vi "START CHECK OUT ITEMS.vi"(11 "REFERENCES":T1) -> ()   [LabVIEW 2019]
uses:
  Controls/References Cluster.ctl
  <vilib>/userDefined/High Color/IMAQdx.ctl
  Controls/Custom Calendar/Custom Calendar.xctl
  <vilib>/Utility/miscctls.llb/LVRowAndColumnTypeDef.ctl
types:
  T1 = typedef "References Cluster.ctl" = cluster{"MAIN PAGES":refnum<vi>, "ADD/EDIT ITEM REFERENCES":cluster{"Identifier":refnum<vi>, "BYU ICN #":refnum<vi>, "Item Description":refnum<vi>, "Comments":refnum<vi>, "Checked Out Date":refnum<vi>, "Due Date":refnum<vi>, "Check Out Location":refnum<vi>, "Reminder Count":refnum<vi>, "Most Recent Reminder Date":refnum<vi>, "BYU ID #":refnum<vi>, "Building/Room":refnum<vi>, "Location in Room":refnum<vi>, "Manual":refnum<vi>, "Manufacturer":refnum<vi>, "Model #":refnum<vi>, "Serial #":refnum<vi>, "Date Acquired":refnum<vi>, "ADD/EDIT ITEM LABEL":refnum<vi>, "ARCHIVE ITEM":refnum<vi>, "Archive Item Inputs":refnum<vi>, "Reminder Notes":refnum<vi>}, "ADD/EDIT USER REFERENCES":cluster{"BYU ID # (##-###-####)":refnum<vi>, "First Name":refnum<vi>, "Last Name":refnum<vi>, "Phone Number (###-###-####)":refnum<vi>, "Email":refnum<vi>, "Department":refnum<vi>, "Graduation Status":refnum<vi>, "Anticipated Graduation Year":refnum<vi>, "Credit Score":refnum<vi>, "Date Added":refnum<vi>, "Graduation Clearance Date":refnum<vi>, "Picture File Name":refnum<vi>, "ADD/EDIT USER LABEL":refnum<vi>, "Department Map":refnum<vi>, "Status Map":refnum<vi>, "Anticipated Graduation Year Map":refnum<vi>, "User Agreement":refnum<vi>, "User Comments":refnum<vi>, "Camera":refnum<vi>}, "RETURN ITEM REFERENCES":cluster{"Item or Person:":refnum<vi>, "Search Return Results":refnum<vi>, "What are you searching for?":refnum<vi>}, "SEARCH DATABASE REFERENCES":cluster{"What to Search For:":refnum<vi>, "Where to Search":refnum<vi>, "Column to Search In":refnum<vi>, "Column to Sort By":refnum<vi>, "Search Database Results":refnum<vi>, "Inventory Column Selector":refnum<vi>, "User Column Selector":refnum<vi>, "Inventory Archive Column Selector":refnum<vi>, "User Archive Column Selector":refnum<vi>, "Sales Tracking Column Selector":refnum<vi>, "Checked In Archive Column Selector":refnum<vi>, "Restore User":refnum<vi>, "Date Range":refnum<vi>, "Dates Less Than":refnum<vi>, "Dates Greater Than":refnum<vi>, "Search Print Receipt":refnum<vi>, "Edit Sale Description":refnum<vi>}, "USER ITEMS REFERENCES":cluster{"USER'S INFORMATION":refnum<vi>, "User's Checked Out Items":refnum<vi>, "User Info Comments":refnum<vi>, "SEE USER INFO COMMENTS":refnum<vi>}, "EDIT ITEMS REFERENCES":cluster{"New Check Out Location":refnum<vi>, "Items to Edit":refnum<vi>, "Edit Items Due Date":refnum<vi>, "New Reminder Notes":refnum<vi>, "New Item Description":refnum<vi>}, "CHECK OUT ITEMS REFERENCES":cluster{"Enter Item:":refnum<vi>, "Check Out Items Due Date":refnum<vi>, "Check Out Location":refnum<vi>, "Items to be Checked Out":refnum<vi>, "Possible Items":refnum<vi>}, "TRANSFER ITEMS REFERENCES":cluster{"Search Parameter":refnum<vi>, "What to Match":refnum<vi>, "Matching Individuals":refnum<vi>, "Items to be Transferred":refnum<vi>}, "SETTINGS REFERENCES":cluster{"PSC Database Settings":refnum<vi>, "PSC Sales Item Spreadsheet":refnum<vi>}, "PSC SALES REFERENCES":cluster{"BYU ID CARD #":refnum<vi>, "Sale Description":refnum<vi>, "Scan or Enter Item Name":refnum<vi>, "Items to be Sold":refnum<vi>, "Grand Total":refnum<vi>, "Item List":refnum<vi>}}
  T2 = typedef "LVRowAndColumnTypeDef.ctl" = cluster{"Row":i32, "Column":i32}
  T3 = enum32{"IDLE", "ADD/EDIT USER", "ADD/EDIT ITEM", "RETURN ITEMS", "SEARCH DATABASE", "USER ITEMS", "CHECK OUT ITEMS", "EDIT ITEMS", "TRANSFER ITEMS", "PSC SALES", "ATRIUM", "INVENTORY TRACKING", "SETTINGS"}
  T4 = cluster{"Enter Item:":refnum<vi>, "Check Out Items Due Date":refnum<vi>, "Check Out Location":refnum<vi>, "Items to be Checked Out":refnum<vi>, "Possible Items":refnum<vi>}
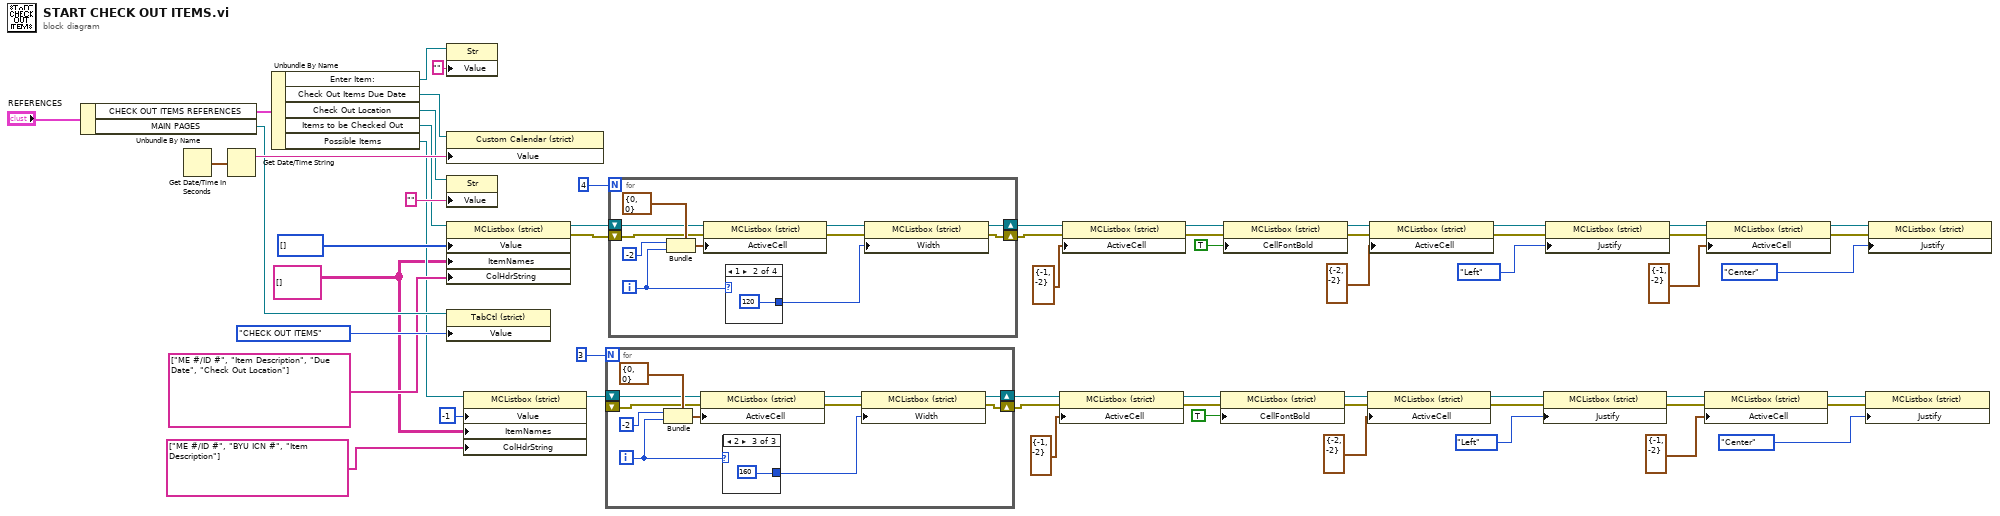
[diagram p0: block diagram]
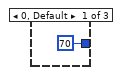
[diagram p2: hidden frame]
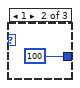
[diagram p3: hidden frame]
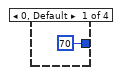
[diagram p4: hidden frame]
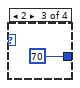
[diagram p5: hidden frame]
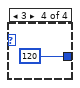
[diagram p6: hidden frame]
diagram:
  w3 = string[][] [] ("Item Names")
  n1 = Unbundle By Name("REFERENCES") -> ("CHECK OUT ITEMS REFERENCES"=w59:T4, "MAIN PAGES"=w49:refnum<vi>)
  n2 = Get Date/Time In Seconds() -> (seconds since 1Jan1904=w55:timestamp)
  n3 = Get Date/Time String(seconds (now)=w55) -> (date string=w54:string)  [unwired: 2 in, 1 out]
  n4 = Unbundle By Name(w59) -> ("Enter Item:"=w58:refnum<vi>, "Check Out Items Due Date"=w56:refnum<vi>, "Check Out Location"=w53:refnum<vi>, "Items to be Checked Out"=w51:refnum<vi>, "Possible Items"=w4:refnum<vi>)
  n5 = property class="Str"(reference=w58, "Value"="") -> ()  [unwired: 1 in, 2 out]
  n6 = property class="Custom Calendar (strict)"(reference=w56, "Value"=w54) -> ()  [unwired: 1 in, 2 out]
  n7 = property class="Str"(reference=w53, "Value"="") -> ()  [unwired: 1 in, 2 out]
  n8 = property class="MCListbox (strict)"(reference=w51, "Value"=i32[] [], "ItemNames"=w3, "ColHdrString"=string[] ["ME #/ID #", "Item Description", "Due Date", "Check Out Location"] ("Column Header Strings[]")) -> (reference out=w46:refnum<vi>, error out=w45:errorcluster)  [unwired: 1 in]
  n9 = property class="TabCtl (strict)"(reference=w49, "Value"=T3."CHECK OUT ITEMS") -> ()  [unwired: 1 in, 2 out]
  n10 = property class="MCListbox (strict)"(reference=w4, "Value"=-1, "ItemNames"=w3, "ColHdrString"=string[] ["ME #/ID #", "BYU ICN #", "Item Description"] ("Column Header Strings[]")) -> (reference out=w5:refnum<vi>)  [unwired: 1 in, 1 out]
  n11 = for {
    N: 3 -> [_]
    shift-right: [w70] -> w24
    shift-left: w5 -> [w67]
    shift-right: [w69] -> w23
    shift-left: _ -> [w66]
    i -> [w63]
    n12 = Bundle(cluster=T2 {"Row"=0, "Column"=0} ("Active Cell:Active Cell"), "Row"=-2, "Column"=w63) -> (w65:T2)
    n13 = property class="MCListbox (strict)"(reference=w67, error in=w66, "ActiveCell"=w65) -> (reference out=w61:refnum<vi>, error out=w60:errorcluster)
    n14 = case shown="2" w63 {
      tunnel: [u32 70 ("Active Cell:Cell Size:Width") u32 100 ("Active Cell:Cell Size:Width") u32 160 ("Active Cell:Cell Size:Width")] -> w62
      frame 0, Default {
      }
      frame 1 {
      }
      frame 2 {
      }
    }
    n15 = property class="MCListbox (strict)"(reference=w61, error in=w60, "Width"=w62) -> (reference out=w70:refnum<vi>, error out=w69:errorcluster)
  }
  n16 = for {
    N: 4 -> [_]
    shift-right: [w84] -> w26
    shift-left: w46 -> [w81]
    shift-right: [w83] -> w27
    shift-left: w45 -> [w80]
    i -> [w77]
    n17 = Bundle(cluster=T2 {"Row"=0, "Column"=0} ("Active Cell:Active Cell"), "Row"=-2, "Column"=w77) -> (w79:T2)
    n18 = property class="MCListbox (strict)"(reference=w81, error in=w80, "ActiveCell"=w79) -> (reference out=w75:refnum<vi>, error out=w74:errorcluster)
    n19 = case shown="1" w77 {
      tunnel: [u32 70 ("Active Cell:Cell Size:Width") u32 120 ("Active Cell:Cell Size:Width") u32 70 ("Active Cell:Cell Size:Width") u32 120 ("Active Cell:Cell Size:Width")] -> w76
      frame 0, Default {
      }
      frame 1 {
      }
      frame 2 {
      }
      frame 3 {
      }
    }
    n20 = property class="MCListbox (strict)"(reference=w75, error in=w74, "Width"=w76) -> (reference out=w84:refnum<vi>, error out=w83:errorcluster)
  }
  n21 = property class="MCListbox (strict)"(reference=w24, error in=w23, "ActiveCell"=T2 {"Row"=-1, "Column"=-2} ("Active Cell:Active Cell")) -> (reference out=w7:refnum<vi>, error out=w8:errorcluster)
  n22 = property class="MCListbox (strict)"(reference=w26, error in=w27, "ActiveCell"=T2 {"Row"=-1, "Column"=-2} ("Active Cell:Active Cell")) -> (reference out=w43:refnum<vi>, error out=w42:errorcluster)
  n23 = property class="MCListbox (strict)"(reference=w7, error in=w8, "CellFontBold"=TRUE ("Active Cell:Cell Font:Bold")) -> (reference out=w10:refnum<vi>, error out=w11:errorcluster)
  n24 = property class="MCListbox (strict)"(reference=w43, error in=w42, "CellFontBold"=TRUE ("Active Cell:Cell Font:Bold")) -> (reference out=w40:refnum<vi>, error out=w39:errorcluster)
  n25 = property class="MCListbox (strict)"(reference=w10, error in=w11, "ActiveCell"=T2 {"Row"=-2, "Column"=-2} ("Active Cell:Active Cell")) -> (reference out=w13:refnum<vi>, error out=w14:errorcluster)
  n26 = property class="MCListbox (strict)"(reference=w40, error in=w39, "ActiveCell"=T2 {"Row"=-2, "Column"=-2} ("Active Cell:Active Cell")) -> (reference out=w37:refnum<vi>, error out=w36:errorcluster)
  n27 = property class="MCListbox (strict)"(reference=w13, error in=w14, "Justify"=enum16{"Left", "Center", "Right"}."Left" ("Active Cell:Cell Justification")) -> (reference out=w18:refnum<vi>, error out=w19:errorcluster)
  n28 = property class="MCListbox (strict)"(reference=w37, error in=w36, "Justify"=enum16{"Left", "Center", "Right"}."Left" ("Active Cell:Cell Justification")) -> (reference out=w32:refnum<vi>, error out=w31:errorcluster)
  n29 = property class="MCListbox (strict)"(reference=w18, error in=w19, "ActiveCell"=T2 {"Row"=-1, "Column"=-2} ("Active Cell:Active Cell")) -> (reference out=w17:refnum<vi>, error out=w16:errorcluster)
  n30 = property class="MCListbox (strict)"(reference=w32, error in=w31, "ActiveCell"=T2 {"Row"=-1, "Column"=-2} ("Active Cell:Active Cell")) -> (reference out=w33:refnum<vi>, error out=w34:errorcluster)
  n31 = property class="MCListbox (strict)"(reference=w17, error in=w16, "Justify"=enum16{"Left", "Center", "Right"}."Center" ("Active Cell:Cell Justification")) -> ()  [unwired: 2 out]
  n32 = property class="MCListbox (strict)"(reference=w33, error in=w34, "Justify"=enum16{"Left", "Center", "Right"}."Center" ("Active Cell:Cell Justification")) -> ()  [unwired: 2 out]
